vi "ProtocolAnalysis.vi"(8 "error in":errorcluster caption="错误输入", 11 "IP":refnum<k5>) -> (0 "error out":errorcluster caption="错误输出", 1 "Disconnected":bool, 3 "IP 2":refnum<k5>)   [LabVIEW 2015]
uses:
  Database_util/Ctl/database_Method.ctl
  Database_util/Ctl/DNS.ctl
  Global/SeverGlobal.vi
  <vilib>/gmath/NI_Gmath.lvlib
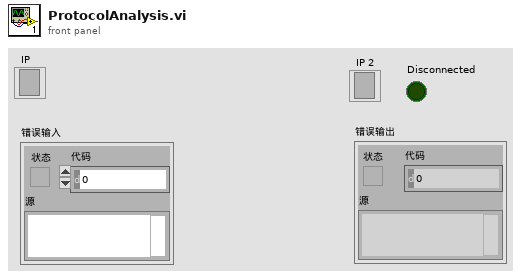
[diagram p1: front panel]
types:
  T1 = typedef "消息头.ctl" = string[]
  T2 = enum16{"Standard", "Buffered", "CRLF", "Immediate"}
  T3 = enum16{"open", "replace", "create", "open or create", "replace or create", "replace or create with confirmation"}
  T4 = typedef "database_Method.ctl" = enum16{"初始化", "查询", "关闭"}
  T5 = typedef "DNS.ctl" = string
  T6 = typedef "响应消息头.ctl" = string
  T7 = cluster{"TCP Ref":refnum<k5>, "IP":string, "userName":string, "A":u16, "COM":u16, "time":u32}[]
  T8 = cluster{"TCP Ref":refnum<k5>, "IP":string, "userName":string, "IN":u16, "OUT":u16, "time":u32}[]
  T9 = cluster{"TCP Ref":refnum<k5>, "Broadcast":refnum<k5>, "TF Ref":refnum<k5>, "IP":string, "port":u16, "userName":string, "passWord":string, "authority":string}[]
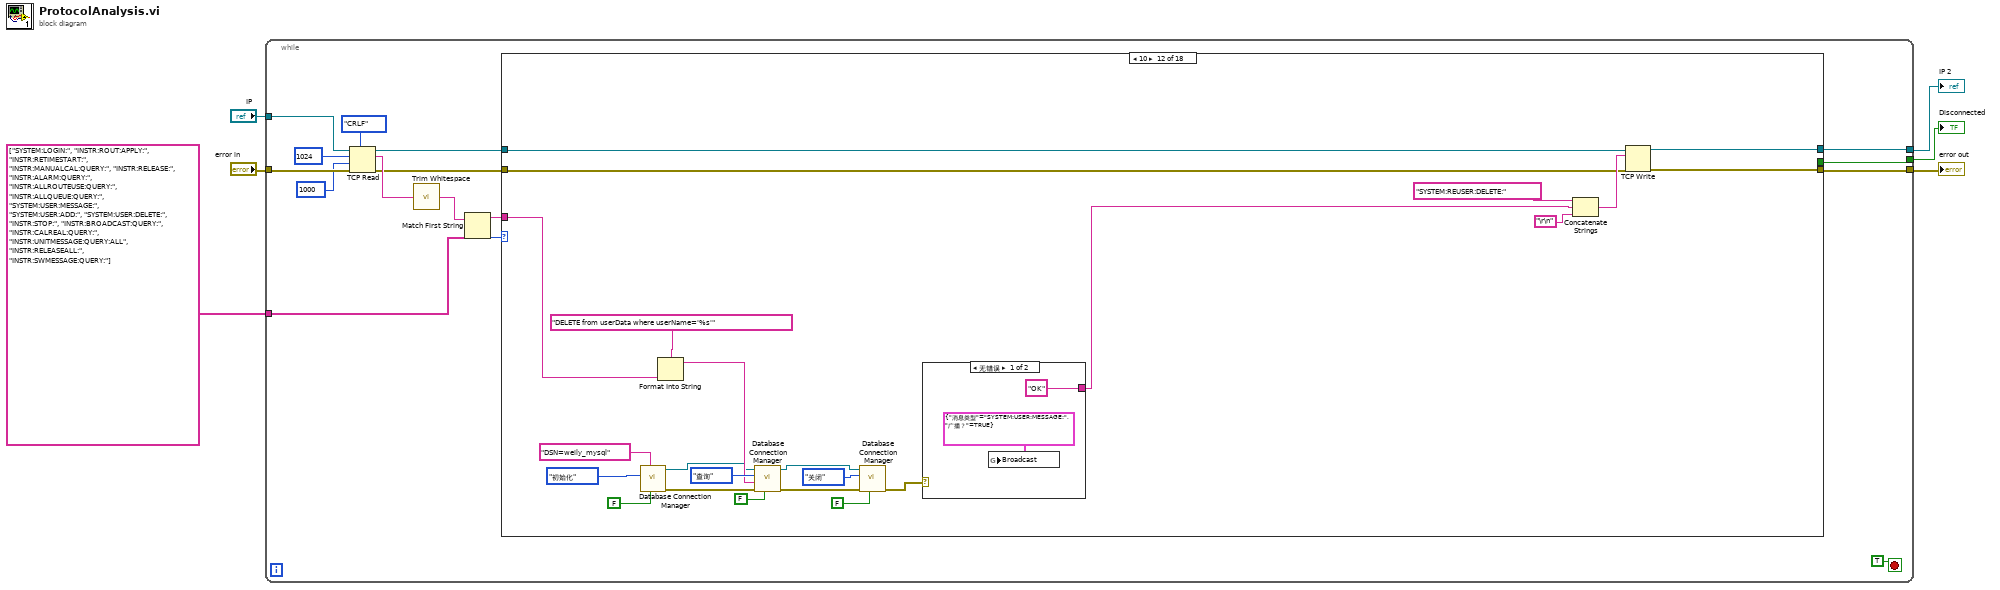
[diagram p0: block diagram]
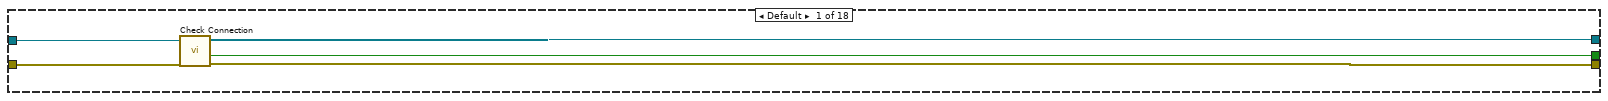
[diagram p2: hidden frame]
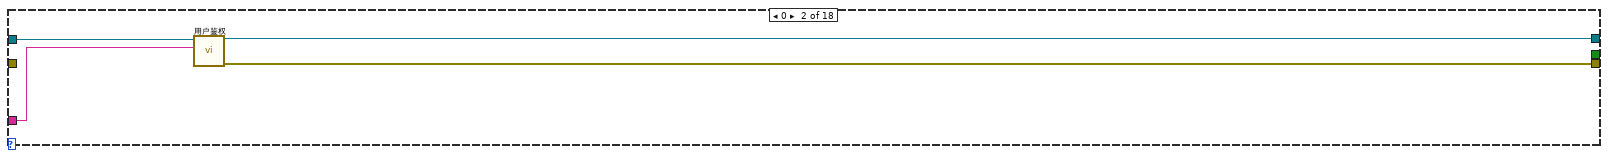
[diagram p3: hidden frame]
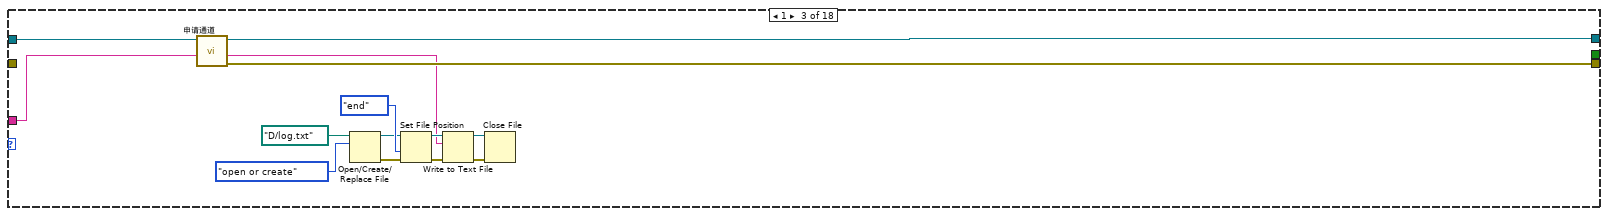
[diagram p4: hidden frame]
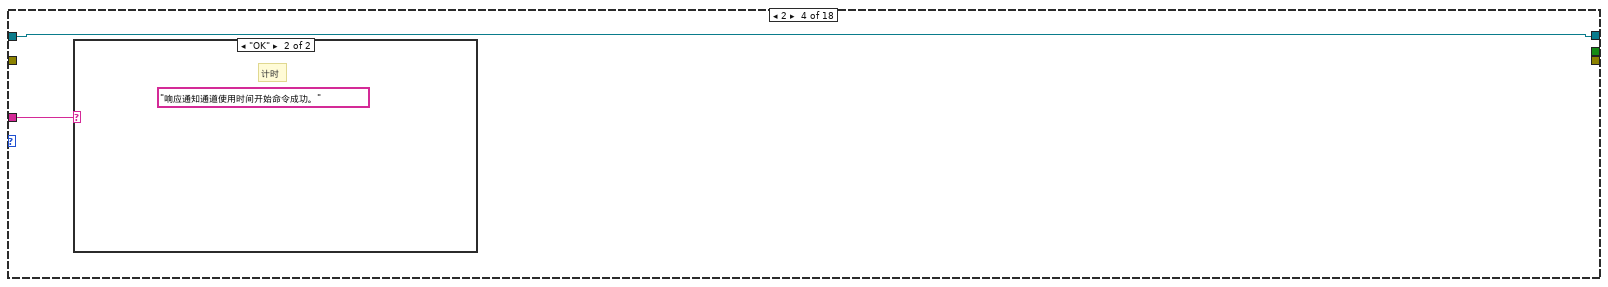
[diagram p5: hidden frame]
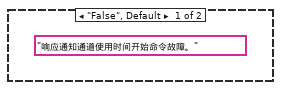
[diagram p6: hidden frame]
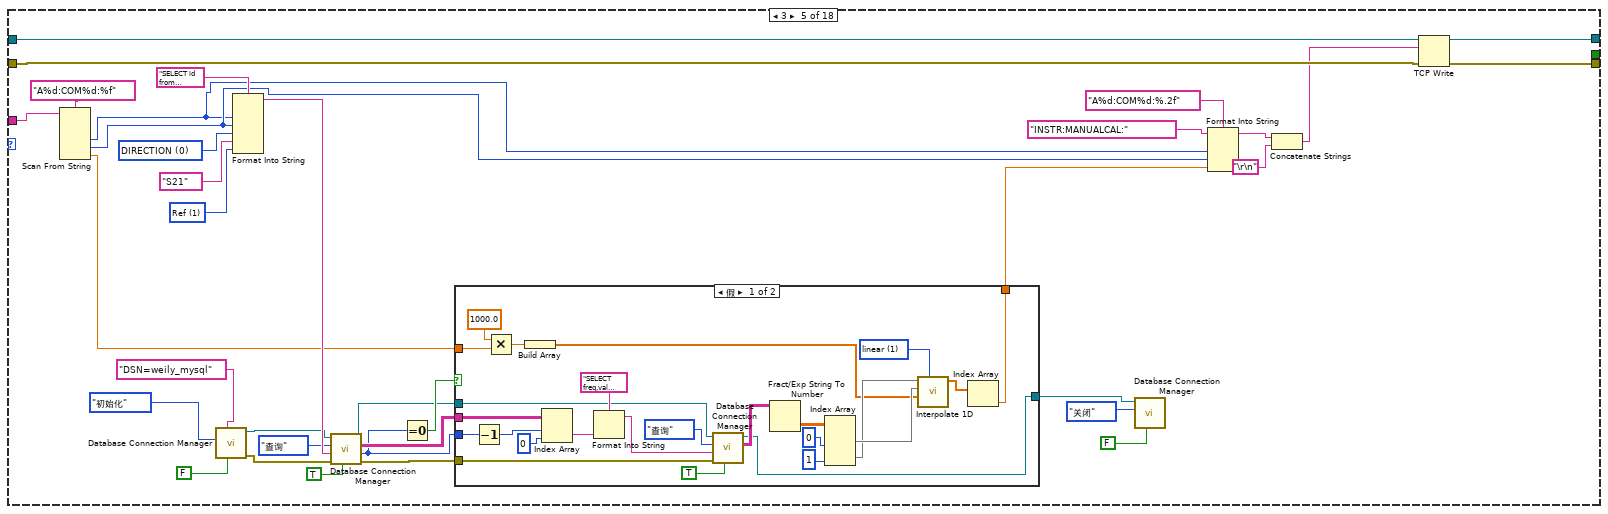
[diagram p7: hidden frame]
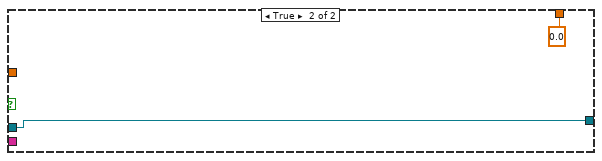
[diagram p8: hidden frame]
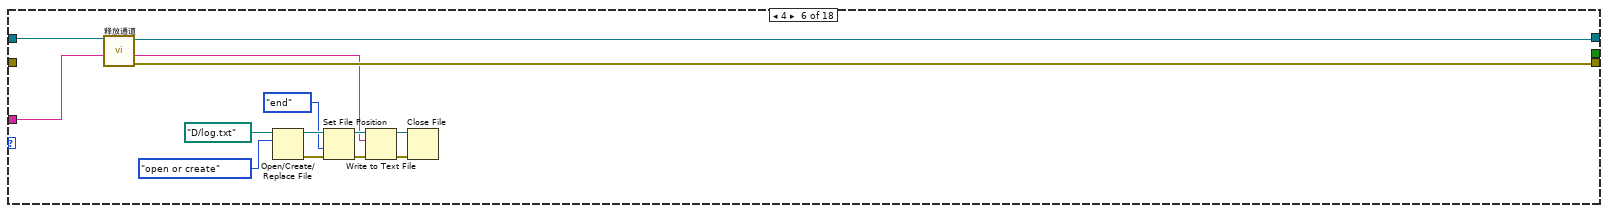
[diagram p9: hidden frame]
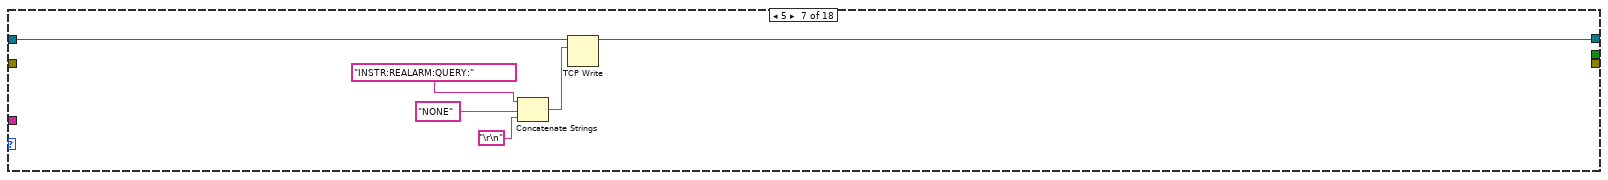
[diagram p10: hidden frame]
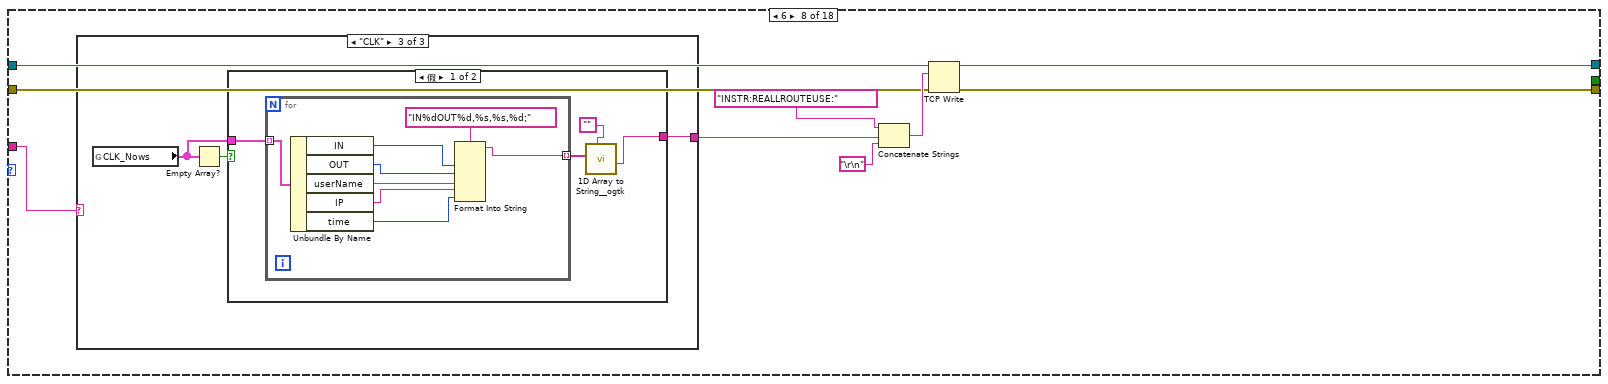
[diagram p11: hidden frame]
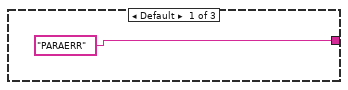
[diagram p12: hidden frame]
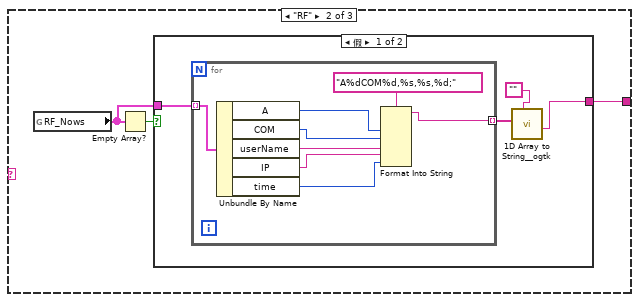
[diagram p13: hidden frame]
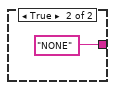
[diagram p14: hidden frame]
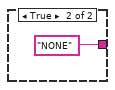
[diagram p15: hidden frame]
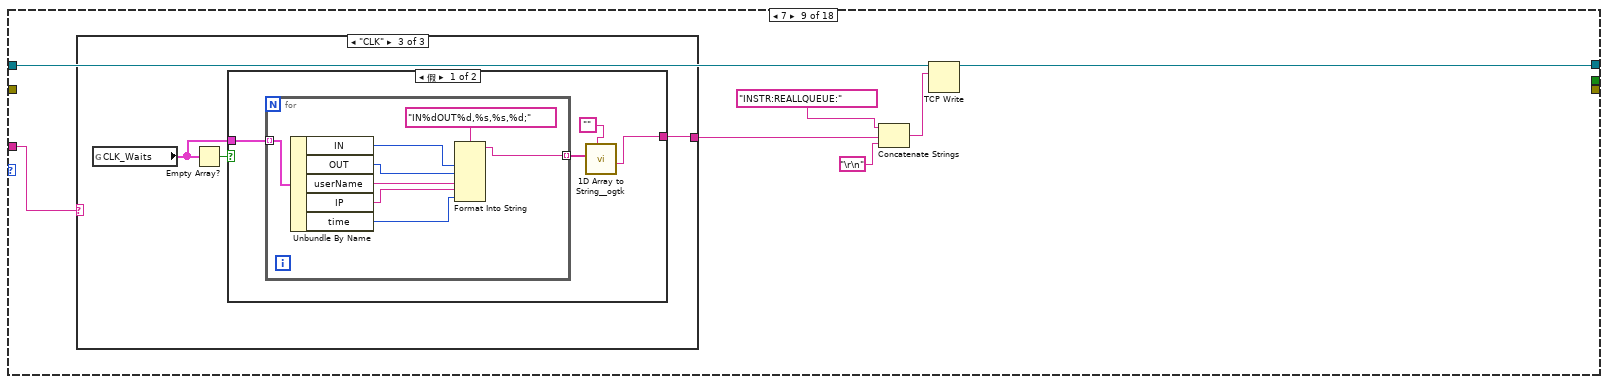
[diagram p16: hidden frame]
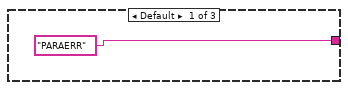
[diagram p17: hidden frame]
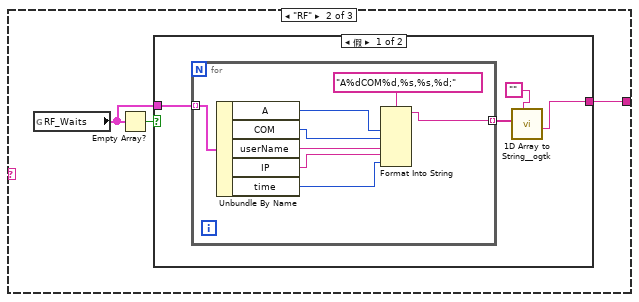
[diagram p18: hidden frame]
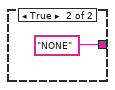
[diagram p19: hidden frame]
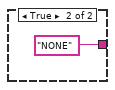
[diagram p20: hidden frame]
diagram:
  n1 = while {
    tunnel: "IP" -> [w21]
    tunnel: [w9] -> w5
    tunnel: [w7] -> w4
    tunnel: "error in" -> [w20]
    tunnel: [w8] -> w2
    tunnel: T1 ["SYSTEM:LOGIN:", "INSTR:ROUT:APPLY:", "INSTR:RETIMESTART:", "INSTR:MANUALCAL:QUERY:", "INSTR:RELEASE:", "INSTR:ALARM:QUERY:", "INSTR:ALLROUTEUSE:QUERY:", "INSTR:ALLQUEUE:QUERY:", "SYSTEM:USER:MESSAGE:", "SYSTEM:USER:ADD:", "SYSTEM:USER:DELETE:", "INSTR:STOP:", "INSTR:BROADCAST:QUERY:", "INSTR:CALREAL:QUERY:", "INSTR:UNITMESSAGE:QUERY:ALL", "INSTR:RELEASEALL:", "INSTR:SWMESSAGE:QUERY:"] ("消息头") -> [w14]
    stop <- TRUE stop-if-true
    n2 = TCP Read(connection ID=w21, bytes to read=1024, error in (no error)=w20, 7:T2."CRLF" ("mode (standard)"), 9:1000 ("timeout ms (25000)")) -> (connection ID out=w13:refnum<k5>, data out=w16:string, error out=w12:errorcluster)
    n3 = call <vilib>:"Trim Whitespace.vi"("string"=w16) -> ("trimmed string"=w15:string)  [unwired: 1 in]
    n4 = Match First String(2:w14, 3:w15) -> (0:w11:i32, 1:w10:string)
    n5 = case shown="10" w11 {
      tunnel: w13 -> [w27 w30 w43 w46 w67 w123 w129 w138 w178 w241 w270 w309 w324 w327 w357 w398 w404 w407]
      tunnel: w12 -> [w26 _ _ _ w66 _ _ w130 _ w240 w269 w308 w323 w326 w360 w397 _ _]
      tunnel: [w25 w29 w42 _ w64 w120 _ w131 _ w232 w271 w310 w321 w326 w359 w400 w402 w405] -> w8
      tunnel: w10 -> [_ w31 w45 w47 w77 w121 _ w133 w173 _ w265 w305 _ _ w375 _ w403 w408]
      tunnel: [w24 w28 w44 w46 w65 w122 w126 w135 w175 w236 w272 w311 w322 w327 w358 w399 w401 w406] -> w9
      tunnel: [w23 _ _ _ _ _ _ _ _ _ _ _ TRUE ("Disconnected") _ _ _ _ _] -> w7
      frame Default {
        n6 = call "Check Connection.vi"("error in (no error)"=w26, "Connection In"=w27) -> ("error out"=w25:errorcluster, "Disconnected"=w23:bool, "Connection out"=w24:refnum<k5>)  [unwired: 7 in]
      }
      frame 0 {
        n7 = call "用户鉴权.vi"("news"=w31, "TCP Network Connection in"=w30) -> ("error out"=w29:errorcluster, "TCP Network Connection out"=w28:refnum<k5>)  [unwired: 8 in]
      }
      frame 1 {
        n8 = call "申请通道.vi"("通道"=w45, "TCP Network Connection in"=w43) -> ("error out"=w42:errorcluster, "ack"=w32:string, "TCP Network Connection out"=w44:refnum<k5>)  [unwired: 7 in]
        n9 = Open/Create/Replace File(file path (use dialog)=path "D:/log.txt" ("文件（使用对话框）"), operation (0:open)=T3."open or create" ("操作(0:open)")) -> (refnum out=w36:refnum<file>, error out=w35:errorcluster)  [unwired: 4 in, 1 out]
        n10 = Set File Position(refnum=w36, from (0:start)=enum16{"start", "end", "current"}."end" ("自（0:起始）"), error in=w35) -> (refnum out=w34:refnum<file>, error out=w33:errorcluster)  [unwired: 1 in]
        n11 = Write to Text File(file (use dialog)=w34, text=w32, error in=w33) -> (refnum out=w38:refnum<file>, error out=w39:errorcluster)  [unwired: 1 in, 1 out]
        n12 = Close File(refnum=w38, error in=w39) -> ()  [unwired: 2 out]
      }
      frame 2 {
        n13 = case shown="\"OK\"" w47 {
          frame "False", Default {
            (unwired) "响应通知通道使用时间开始命令故障。" ("message")
          }
          frame "OK" {
            (unwired) "响应通知通道使用时间开始命令成功。" ("message")
            # "计时"
          }
        }
      }
      frame 3 {
        w79 = u16 1 items=["noRef", "Ref"] ("Ref")
        w81 = u16 0 items=["DIRECTION", "CALIBRATION"] ("TESTTYPE")
        n14 = Scan From String(format string="A%d:COM%d:%f", input string=w77) -> (output 1=w60:i32, output 2=w61:i32, output 3=w68:dbl)  [unwired: 5 in, 3 out]
        n15 = call "Database Connection Manager.vi"("Return Data (T)"=FALSE, "ConnectionString"=T5 "DSN=weily_mysql", "Method"=database_Method."初始化") -> ("error out"=w51:errorcluster, "ADODB._Connection Out"=w52:refnum<k7>)  [unwired: 5 in, 2 out]
        n16 = Format Into String(format string="SELECT id from testData where portIn=%d AND portOut=%d AND testType=%d AND updateType='%s' AND unitType=%d" ("String"), w60, w61, w81, "S21" ("S-Parameter"), w79) -> (resulting string=w75:string)  [unwired: 2 in, 1 out]
        n17 = call "Database Connection Manager.vi"("Return Data (T)"=TRUE, "error in (no error)"=w51, "Command Text"=w75, "Method"=database_Method."查询", "ADODB._Connection In"=w52) -> ("error out"=w70:errorcluster, "Rows Fetched"=w71:i32, "Data"=w72:string[][], "ADODB._Connection Out"=w69:refnum<k7>)  [unwired: 3 in]
        n18 = Equal To 0?(x=w71) -> (x = 0?=w73:bool)
        n19 = case shown="假" w73 {
          tunnel: w70 -> [w98 _]
          tunnel: w72 -> [w104 _]
          tunnel: w71 -> [w102 _]
          tunnel: w69 -> [w99 w108]
          tunnel: w68 -> [w96 _]
          tunnel: [w85 0.0 ("Numeric")] -> w59
          tunnel: [w83 w108] -> w49
          frame False {
            w89 = 1 items=["nearest", "linear", "spline", "cubic Hermite", "Lagrange"] ("method")
            n20 = Decrement(x=w102) -> (x-1=w107:i32)
            n21 = Multiply(x=1000.0, y=w96) -> (x*y=w94:dbl)
            n22 = Build Array(w94) -> (w86:dbl[])
            n23 = Index Array(array=w104, index (row)=w107, index (col)=0) -> (element=w103:string)
            n24 = Format Into String(format string="SELECT freq,val from microwaveData where pid=%s" ("String"), w103) -> (resulting string=w97:string)  [unwired: 2 in, 1 out]
            n25 = call "Database Connection Manager.vi"("Return Data (T)"=TRUE, "error in (no error)"=w98, "Command Text"=w97, "Method"=database_Method."查询", "ADODB._Connection In"=w99) -> ("Data"=w93:string[][], "ADODB._Connection Out"=w83:refnum<k7>)  [unwired: 3 in, 2 out]
            n26 = Fract/Exp String To Number(string=w93) -> (number=w92:dbl[][])  [unwired: 3 in, 1 out]
            n27 = Index Array(array=w92, index (col) #1=0 ("index (row)"), index (col) #2=1 ("index (row)")) -> (element #1=w88:dbl[], element #2=w87:dbl[])  [unwired: 2 in]
            n28 = call <vilib>:"Interpolate 1D.vi"("method"=w89, "xi"=w86, "X"=w88, "Y"=w87) -> ("yi"=w84:dbl[])  [unwired: 5 in, 2 out]
            n29 = Index Array(array=w84) -> (element=w85:dbl)  [unwired: 1 in]
          }
          frame True {
          }
        }
        n30 = call "Database Connection Manager.vi"("Return Data (T)"=FALSE, "Method"=database_Method."关闭", "ADODB._Connection In"=w49) -> ()  [unwired: 5 in, 4 out]
        n31 = Format Into String(format string="A%d:COM%d:%.2f", initial string=T6 "INSTR:MANUALCAL:" ("Combo Box"), w60, w61, w59) -> (resulting string=w58:string)  [unwired: 1 in, 1 out]
        n32 = Concatenate Strings(w58, "\r\n") -> (w56:string)
        n33 = TCP Write(connection ID=w67, data in=w56, error in (no error)=w66) -> (connection ID out=w65:refnum<k5>, error out=w64:errorcluster)  [unwired: 1 in, 1 out]
      }
      frame 4 {
        n34 = call "释放通道.vi"("通道"=w121, "TCP Network Connection in"=w123) -> ("error out"=w120:errorcluster, "ack"=w111:string, "TCP Network Connection out"=w122:refnum<k5>)  [unwired: 7 in]
        n35 = Open/Create/Replace File(file path (use dialog)=path "D:/log.txt" ("文件（使用对话框）"), operation (0:open)=T3."open or create" ("操作(0:open)")) -> (refnum out=w115:refnum<file>, error out=w114:errorcluster)  [unwired: 4 in, 1 out]
        n36 = Set File Position(refnum=w115, from (0:start)=enum16{"start", "end", "current"}."end" ("自（0:起始）"), error in=w114) -> (refnum out=w113:refnum<file>, error out=w112:errorcluster)  [unwired: 1 in]
        n37 = Write to Text File(file (use dialog)=w113, text=w111, error in=w112) -> (refnum out=w116:refnum<file>, error out=w117:errorcluster)  [unwired: 1 in, 1 out]
        n38 = Close File(refnum=w116, error in=w117) -> ()  [unwired: 2 out]
      }
      frame 5 {
        n39 = Concatenate Strings(T6 "INSTR:REALARM:QUERY:" ("Combo Box"), "NONE" ("string"), "\r\n") -> (w125:string)
        n40 = TCP Write(connection ID=w129, data in=w125) -> (connection ID out=w126:refnum<k5>)  [unwired: 2 in, 2 out]
      }
      frame 6 {
        n41 = case shown="\"CLK\"" w133 {
          tunnel: ["PARAERR" ("string") w141 w156] -> w132
          frame Default {
          }
          frame "RF" {
            n42 = global read "SeverGlobal.vi" "RF_Nows"() -> (w140:T7)
            n43 = Empty Array?(array=w140) -> (empty?=w142:bool)
            n44 = case shown="假" w142 {
              tunnel: [w143 "NONE" ("string")] -> w141
              tunnel: w140 -> [w146 _]
              frame False {
                n45 = for {
                  tunnel: w146 -> [w154] mode=indexing
                  tunnel: [w147] -> w145 mode=indexing
                  n46 = Unbundle By Name(w154) -> ("A"=w152:u16, "COM"=w151:u16, "userName"=w150:string, "IP"=w149:string, "time"=w148:u32)
                  n47 = Format Into String(format string="A%dCOM%d,%s,%s,%d;", w152, w151, w150, w149, w148) -> (resulting string=w147:string)  [unwired: 2 in, 1 out]
                }
                n48 = call <userlib>:"1D Array to String__ogtk.vi"("delimiter (Tab)"="", "Array of Strings"=w145) -> ("delimited string"=w143:string)  [unwired: 9 in]
              }
              frame True {
              }
            }
          }
          frame "CLK" {
            n49 = global read "SeverGlobal.vi" "CLK_Nows"() -> (w157:T8)
            n50 = Empty Array?(array=w157) -> (empty?=w158:bool)
            n51 = case shown="假" w158 {
              tunnel: [w159 "NONE" ("string")] -> w156
              tunnel: w157 -> [w162 _]
              frame False {
                n52 = for {
                  tunnel: w162 -> [w170] mode=indexing
                  tunnel: [w163] -> w161 mode=indexing
                  n53 = Unbundle By Name(w170) -> ("IN"=w168:u16, "OUT"=w167:u16, "userName"=w166:string, "IP"=w165:string, "time"=w164:u32)
                  n54 = Format Into String(format string="IN%dOUT%d,%s,%s,%d;", w168, w167, w166, w165, w164) -> (resulting string=w163:string)  [unwired: 2 in, 1 out]
                }
                n55 = call <userlib>:"1D Array to String__ogtk.vi"("delimiter (Tab)"="", "Array of Strings"=w161) -> ("delimited string"=w159:string)  [unwired: 9 in]
              }
              frame True {
              }
            }
          }
        }
        n56 = Concatenate Strings(T6 "INSTR:REALLROUTEUSE:" ("Combo Box"), w132, "\r\n") -> (w134:string)
        n57 = TCP Write(connection ID=w138, data in=w134, error in (no error)=w130) -> (connection ID out=w135:refnum<k5>, error out=w131:errorcluster)  [unwired: 1 in, 1 out]
      }
      frame 7 {
        n58 = case shown="\"CLK\"" w173 {
          tunnel: ["PARAERR" ("string") w181 w196] -> w172
          frame Default {
          }
          frame "RF" {
            n59 = global read "SeverGlobal.vi" "RF_Waits"() -> (w180:T7)
            n60 = Empty Array?(array=w180) -> (empty?=w182:bool)
            n61 = case shown="假" w182 {
              tunnel: [w183 "NONE" ("string")] -> w181
              tunnel: w180 -> [w186 _]
              frame False {
                n62 = for {
                  tunnel: w186 -> [w194] mode=indexing
                  tunnel: [w187] -> w185 mode=indexing
                  n63 = Unbundle By Name(w194) -> ("A"=w192:u16, "COM"=w191:u16, "userName"=w190:string, "IP"=w189:string, "time"=w188:u32)
                  n64 = Format Into String(format string="A%dCOM%d,%s,%s,%d;", w192, w191, w190, w189, w188) -> (resulting string=w187:string)  [unwired: 2 in, 1 out]
                }
                n65 = call <userlib>:"1D Array to String__ogtk.vi"("delimiter (Tab)"="", "Array of Strings"=w185) -> ("delimited string"=w183:string)  [unwired: 9 in]
              }
              frame True {
              }
            }
          }
          frame "CLK" {
            n66 = global read "SeverGlobal.vi" "CLK_Waits"() -> (w197:T8)
            n67 = Empty Array?(array=w197) -> (empty?=w198:bool)
            n68 = case shown="假" w198 {
              tunnel: [w199 "NONE" ("string")] -> w196
              tunnel: w197 -> [w202 _]
              frame False {
                n69 = for {
                  tunnel: w202 -> [w210] mode=indexing
                  tunnel: [w203] -> w201 mode=indexing
                  n70 = Unbundle By Name(w210) -> ("IN"=w208:u16, "OUT"=w207:u16, "userName"=w206:string, "IP"=w205:string, "time"=w204:u32)
                  n71 = Format Into String(format string="IN%dOUT%d,%s,%s,%d;", w208, w207, w206, w205, w204) -> (resulting string=w203:string)  [unwired: 2 in, 1 out]
                }
                n72 = call <userlib>:"1D Array to String__ogtk.vi"("delimiter (Tab)"="", "Array of Strings"=w201) -> ("delimited string"=w199:string)  [unwired: 9 in]
              }
              frame True {
              }
            }
          }
        }
        n73 = Concatenate Strings(T6 "INSTR:REALLQUEUE:" ("Combo Box"), w172, "\r\n") -> (w174:string)
        n74 = TCP Write(connection ID=w178, data in=w174) -> (connection ID out=w175:refnum<k5>)  [unwired: 2 in, 2 out]
      }
      frame 8 {
        n75 = global read "SeverGlobal.vi" "Clients"() -> (w239:T9)
        n76 = for {
          tunnel: w239 -> [w252] mode=indexing
          tunnel: [w245] -> w227 mode=indexing
          n77 = Unbundle By Name(w252) -> ("userName"=w250:string, "passWord"=w249:string, "IP"=w248:string, "port"=w247:u16, "authority"=w246:string)
          n78 = Format Into String(format string="%s:%s:%s:%d:%s", w250, w249, w248, w247, w246) -> (resulting string=w245:string)  [unwired: 2 in, 1 out]
        }
        n79 = call "Database Connection Manager.vi"("Return Data (T)"=FALSE, "ConnectionString"=T5 "DSN=weily_mysql", "Method"=database_Method."初始化") -> ("error out"=w216:errorcluster, "ADODB._Connection Out"=w219:refnum<k7>)  [unwired: 5 in, 2 out]
        n80 = call <userlib>:"1D Array to String__ogtk.vi"("delimiter (Tab)"=";", "Array of Strings"=w227) -> ("delimited string"=w225:string)  [unwired: 9 in]
        n81 = call "Database Connection Manager.vi"("Return Data (T)"=TRUE, "error in (no error)"=w216, "Command Text"="SELECT userName,password,authority FROM userData" ("SQL"), "Method"=database_Method."查询", "ADODB._Connection In"=w219) -> ("error out"=w212:errorcluster, "Data"=w224:string[][], "ADODB._Connection Out"=w213:refnum<k7>)  [unwired: 3 in, 1 out]
        n82 = for {
          tunnel: w224 -> [w244] mode=indexing
          tunnel: [w242] -> w223 mode=indexing
          n83 = call <userlib>:"1D Array to String__ogtk.vi"("delimiter (Tab)"=":", "Array of Strings"=w244) -> ("delimited string"=w242:string)  [unwired: 9 in]
        }
        n84 = call "Database Connection Manager.vi"("Return Data (T)"=FALSE, "error in (no error)"=w212, "Method"=database_Method."关闭", "ADODB._Connection In"=w213) -> ()  [unwired: 4 in, 4 out]
        n85 = call <userlib>:"1D Array to String__ogtk.vi"("delimiter (Tab)"="$", "Array of Strings"=w223) -> ("delimited string"=w221:string)  [unwired: 9 in]
        n86 = global read "SeverGlobal.vi" "memebers"() -> (w230:i32)
        n87 = Format Into String(format string="%s&%s&%d", w225, w221, w230) -> (resulting string=w228:string)  [unwired: 2 in, 1 out]
        n88 = Concatenate Strings("SYSTEM:REUSER:MESSAGE:", w228, "\r\n") -> (w237:string)
        n89 = TCP Write(connection ID=w241, data in=w237, error in (no error)=w240) -> (connection ID out=w236:refnum<k5>, error out=w232:errorcluster)  [unwired: 1 in, 1 out]
      }
      frame 9 {
        n90 = call <userlib>:"String to 1D Array__ogtk.vi"("delimiter (Tab)"=":", "string"=w265) -> ("Array of Strings"=w266:string[])  [unwired: 9 in]
        n91 = Index Array(array=w266) -> (element #1=w263:string, element #2=w262:string, element #3=w261:string)  [unwired: 3 in]
        n92 = call "Database Connection Manager.vi"("Return Data (T)"=FALSE, "ConnectionString"=T5 "DSN=weily_mysql", "Method"=database_Method."初始化") -> ("error out"=w257:errorcluster, "ADODB._Connection Out"=w258:refnum<k7>)  [unwired: 5 in, 2 out]
        n93 = Format Into String(format string="SELECT * from userData where isDeled=0 AND userName='%s'" ("SQL"), w263) -> (resulting string=w278:string)  [unwired: 2 in, 1 out]
        n94 = call "Database Connection Manager.vi"("Return Data (T)"=TRUE, "error in (no error)"=w257, "Command Text"=w278, "Method"=database_Method."查询", "ADODB._Connection In"=w258) -> ("Rows Fetched"=w277:i32, "ADODB._Connection Out"=w275:refnum<k7>)  [unwired: 3 in, 2 out]
        n95 = Equal To 0?(x=w277) -> (x = 0?=w276:bool)
        n96 = case shown="真" w276 {
          tunnel: ["REPEAT" ("消息") "OK" ("消息")] -> w267
          tunnel: w275 -> [w282 w292]
          tunnel: w261 -> [_ w289]
          tunnel: w262 -> [_ w288]
          tunnel: w263 -> [_ w287]
          tunnel: [w282 w284] -> w253
          frame False {
          }
          frame True {
            n97 = Format Into String(format string="INSERT INTO userData (username,password,authority) values('%s','%s','%s')" ("SQL"), w287, w288, w289) -> (resulting string=w286:string)  [unwired: 2 in, 1 out]
            n98 = call "Database Connection Manager.vi"("Return Data (T)"=FALSE, "Command Text"=w286, "Method"=database_Method."查询", "ADODB._Connection In"=w292) -> ("ADODB._Connection Out"=w284:refnum<k7>)  [unwired: 4 in, 3 out]
            n99 = global write "SeverGlobal.vi" "Broadcast"(cluster{"消息类型":string, "广播？":bool} {"消息类型"="SYSTEM:USER:MESSAGE:", "广播？"=TRUE} ("Broadcast")) -> ()
          }
        }
        n100 = call "Database Connection Manager.vi"("Return Data (T)"=FALSE, "Method"=database_Method."关闭", "ADODB._Connection In"=w253) -> ()  [unwired: 5 in, 4 out]
        n101 = Concatenate Strings("SYSTEM:REUSER:ADD:", w267, "\r\n") -> (w274:string)
        n102 = TCP Write(connection ID=w270, data in=w274, error in (no error)=w269) -> (connection ID out=w272:refnum<k5>, error out=w271:errorcluster)  [unwired: 1 in, 1 out]
      }
      frame 10 {
        n103 = call "Database Connection Manager.vi"("Return Data (T)"=FALSE, "ConnectionString"=T5 "DSN=weily_mysql", "Method"=database_Method."初始化") -> ("error out"=w300:errorcluster, "ADODB._Connection Out"=w301:refnum<k7>)  [unwired: 5 in, 2 out]
        n104 = Format Into String(format string="DELETE from userData where userName='%s'" ("SQL"), w305) -> (resulting string=w314:string)  [unwired: 2 in, 1 out]
        n105 = call "Database Connection Manager.vi"("Return Data (T)"=FALSE, "error in (no error)"=w300, "Command Text"=w314, "Method"=database_Method."查询", "ADODB._Connection In"=w301) -> ("error out"=w295:errorcluster, "ADODB._Connection Out"=w297:refnum<k7>)  [unwired: 3 in, 2 out]
        n106 = call "Database Connection Manager.vi"("Return Data (T)"=FALSE, "error in (no error)"=w295, "Method"=database_Method."关闭", "ADODB._Connection In"=w297) -> ("error out"=w296:errorcluster)  [unwired: 4 in, 3 out]
        n107 = case shown="无错误" w296 {
          tunnel: ["OK" ("消息") "FAIL" ("消息")] -> w306
          frame No Error {
            n108 = global write "SeverGlobal.vi" "Broadcast"(cluster{"消息类型":string, "广播？":bool} {"消息类型"="SYSTEM:USER:MESSAGE:", "广播？"=TRUE} ("Broadcast")) -> ()
          }
          frame Error {
          }
        }
        n109 = Concatenate Strings("SYSTEM:REUSER:DELETE:", w306, "\r\n") -> (w313:string)
        n110 = TCP Write(connection ID=w309, data in=w313, error in (no error)=w308) -> (connection ID out=w311:refnum<k5>, error out=w310:errorcluster)  [unwired: 1 in, 1 out]
      }
      frame 11 {
        n111 = call "Handle after Disconnection.vi"("error in (no error)"=w323, "Connection In"=w324) -> ("error out"=w321:errorcluster, "Connection out"=w322:refnum<k5>)  [unwired: 8 in]
      }
      frame 12 {
        n112 = stacked-sequence {
          frame #0 {
            n113 = Bundle("INSTR:ALLROUTE:RF", TRUE) -> (w329:cluster{string, bool})  [unwired: 1 in]
            n114 = global write "SeverGlobal.vi" "Broadcast"(w329) -> ()
            n115 = Wait (ms)(milliseconds to wait=u32 20) -> ()  [unwired: 1 out]
          }
          frame #1 {
            n116 = Bundle("INSTR:ALLROUTE:CLK", TRUE) -> (w333:cluster{string, bool})  [unwired: 1 in]
            n117 = global write "SeverGlobal.vi" "Broadcast"(w333) -> ()
            n118 = Wait (ms)(milliseconds to wait=u32 20) -> ()  [unwired: 1 out]
          }
          frame #2 {
            n119 = Bundle("SYSTEM:USER:MESSAGE:", TRUE) -> (w339:cluster{string, bool})  [unwired: 1 in]
            n120 = global write "SeverGlobal.vi" "Broadcast"(w339) -> ()
            n121 = Wait (ms)(milliseconds to wait=u32 20) -> ()  [unwired: 1 out]
          }
          frame #3 {
            n122 = Bundle("", FALSE) -> (w342:cluster{string, bool})  [unwired: 1 in]
            n123 = global write "SeverGlobal.vi" "Broadcast"(w342) -> ()
          }
        }
      }
      frame 13 {
        w369 = u16 1 items=["noRef", "Ref"] ("Ref")
        w371 = u16 0 items=["DIRECTION", "CALIBRATION"] ("TESTTYPE")
        n124 = Scan From String(format string="A%d:COM%d", input string=w375) -> (output 1=w353:i32, output 2=w352:i32)  [unwired: 4 in, 3 out]
        n125 = call "Database Connection Manager.vi"("Return Data (T)"=FALSE, "ConnectionString"=T5 "DSN=weily_mysql", "Method"=database_Method."初始化") -> ("error out"=w344:errorcluster, "ADODB._Connection Out"=w345:refnum<k7>)  [unwired: 5 in, 2 out]
        n126 = Format Into String(format string="SELECT id from testData where portIn=%d AND portOut=%d AND testType=%d AND updateType='%s' AND unitType=%d" ("String"), w353, w352, w371, "S21" ("S-Parameter"), w369) -> (resulting string=w368:string)  [unwired: 2 in, 1 out]
        n127 = call "Database Connection Manager.vi"("Return Data (T)"=TRUE, "error in (no error)"=w344, "Command Text"=w368, "Method"=database_Method."查询", "ADODB._Connection In"=w345) -> ("Rows Fetched"=w365:i32, "Data"=w366:string[][], "ADODB._Connection Out"=w363:refnum<k7>)  [unwired: 3 in, 1 out]
        n128 = Equal To 0?(x=w365) -> (x = 0?=w364:bool)
        n129 = case shown="假" w364 {
          tunnel: w366 -> [w389 _]
          tunnel: w365 -> [w388 _]
          tunnel: w363 -> [w385 w395]
          tunnel: [w378 "NULL" ("spreadsheet string")] -> w351
          tunnel: [w376 w395] -> w343
          frame False {
            n130 = Decrement(x=w388) -> (x-1=w390:i32)
            n131 = Index Array(array=w389, index (row)=w390, index (col)=0) -> (element=w386:string)
            n132 = Format Into String(format string="SELECT freq,val from microwaveData where pid=%s" ("String"), w386) -> (resulting string=w383:string)  [unwired: 2 in, 1 out]
            n133 = call "Database Connection Manager.vi"("Return Data (T)"=TRUE, "Command Text"=w383, "Method"=database_Method."查询", "ADODB._Connection In"=w385) -> ("Data"=w379:string[][], "ADODB._Connection Out"=w376:refnum<k7>)  [unwired: 4 in, 2 out]
            n134 = Transpose 2D Array(2D array=w379) -> (transposed array=w377:string[][])
            n135 = for {
              tunnel: w377 -> [w394] mode=indexing
              tunnel: [w392] -> w381 mode=indexing
              n136 = call <userlib>:"1D Array to String__ogtk.vi"("delimiter (Tab)"="&", "Array of Strings"=w394) -> ("delimited string"=w392:string)  [unwired: 9 in]
            }
            n137 = call <userlib>:"1D Array to String__ogtk.vi"("delimiter (Tab)"="$", "Array of Strings"=w381) -> ("delimited string"=w378:string)  [unwired: 9 in]
          }
          frame True {
          }
        }
        n138 = call "Database Connection Manager.vi"("Return Data (T)"=FALSE, "Method"=database_Method."关闭", "ADODB._Connection In"=w343) -> ()  [unwired: 5 in, 4 out]
        n139 = Format Into String(format string="A%d:COM%d:%s", initial string="INSTR:CALREAL:REQUERY:", w353, w352, w351) -> (resulting string=w355:string)  [unwired: 1 in, 1 out]
        n140 = Concatenate Strings(w355, "\r\n") -> (w362:string)
        n141 = TCP Write(connection ID=w357, data in=w362, error in (no error)=w360) -> (connection ID out=w358:refnum<k5>, error out=w359:errorcluster)  [unwired: 1 in, 1 out]
      }
      frame 14 {
        n142 = call "查询温度风扇.vi"("error in (no error)"=w397, "TCP Network Connection in"=w398) -> ("error out"=w400:errorcluster, "TCP Network Connection out"=w399:refnum<k5>)  [unwired: 8 in]
      }
      frame 15 {
        n143 = call "释放所有通道.vi"("RF/CLK"=w403, "TCP Network Connection in"=w404) -> ("error out"=w402:errorcluster, "TCP Network Connection out"=w401:refnum<k5>)  [unwired: 8 in]
      }
      frame 16 {
        n144 = call "查询开关信息.vi"("NEWS"=w408, "TCP Network Connection in"=w407) -> ("error out"=w405:errorcluster, "TCP Network Connection out"=w406:refnum<k5>)  [unwired: 8 in]
      }
    }
  }
  "error out" <- w2
  "IP 2" <- w5
  "Disconnected" <- w4
